vi "json Parse core.vi"(8 "error in (no error)":errorcluster, 9 "default":variant, 10 "path":string, 11 "JSON Document in":refnum<class "JSON Document.lvclass">) -> (0 "error out":errorcluster, 1 "defaulted paths":string[](array[string]), 2 "value":variant, 3 "JSON Document out":refnum<class "JSON Document.lvclass">)   [LabVIEW 2016, in "JSON Document.lvclass"]
uses:
  JSON Document.lvclass
  <vilib>/Utility/Data Type/NI_Data Type.lvlib
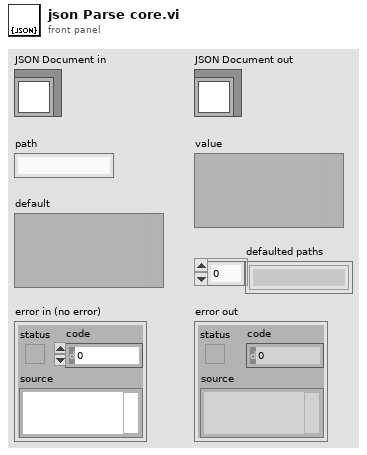
[diagram p1: front panel]
types:
  T1 = typedef "NI_Data Type.lvlib/Data Type.ctl" = enum8{"Invalid Type", "Void", "I8", "I16", "I32", "I64", "U8", "U16", "U32", "U64", "Single Float", "Double Float", "Extended Float", "Single Complex", "Double Complex", "Extended Complex", "Enum U8", "Enum U16", "Enum U32", "Enum U64", "Single Float With Unit", "Double Float With Unit", "Extended Float With Unit", "Single Complex with Unit", "Double Complex with Unit", "Extended Complex with Unit", "Boolean", "String", "Path", "Picture", "Tag", "Array", "Cluster", "Variant", "LV Variant", "Waveform", "Timestamp", "Digital Waveform", "Digital Data", "ExpressData", "Refnum", "External Data", "VI", "Poly VI", "LabVIEW Class Instance", "Fixed Point"}
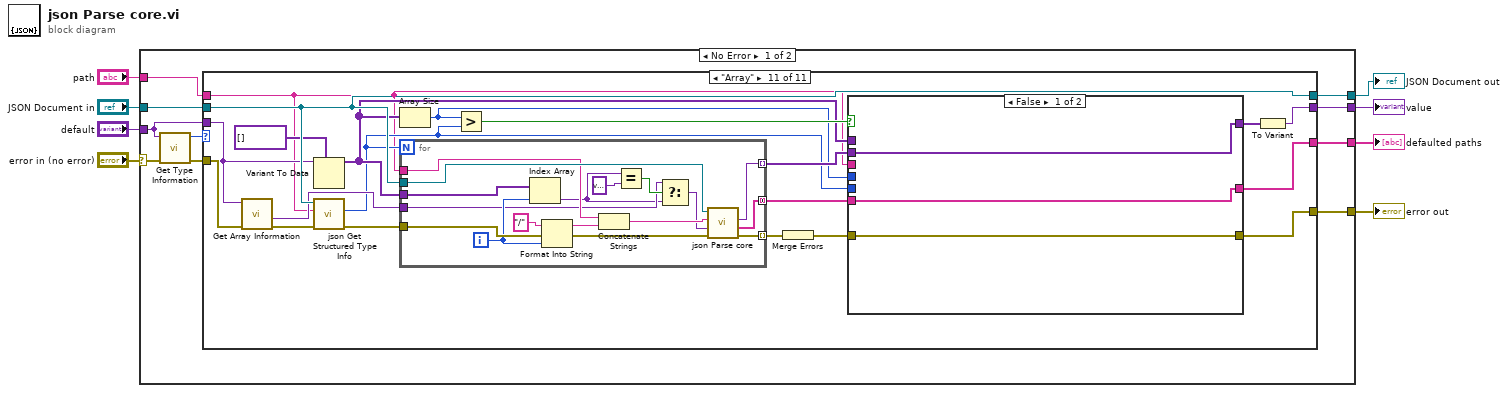
[diagram p0: block diagram]
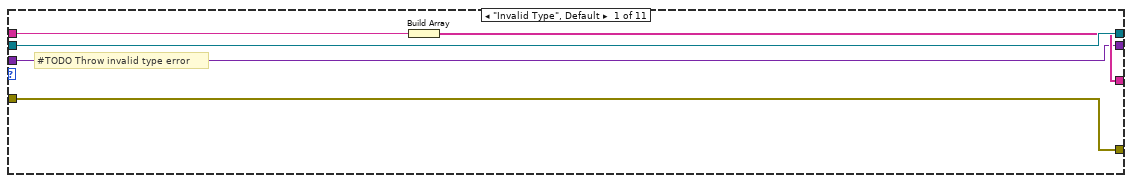
[diagram p2: hidden frame]
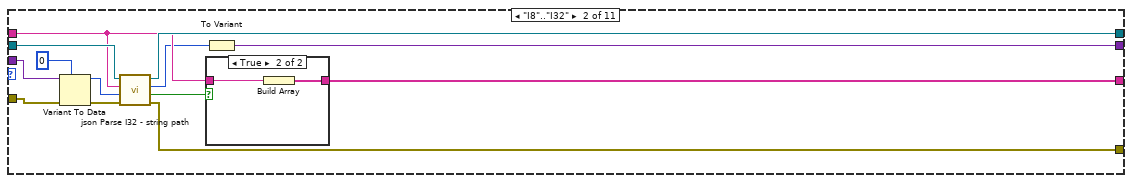
[diagram p3: hidden frame]
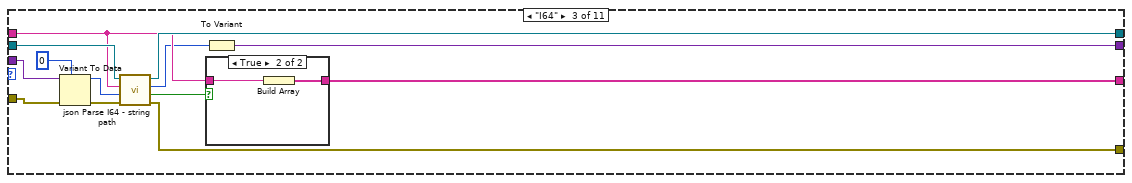
[diagram p5: hidden frame]
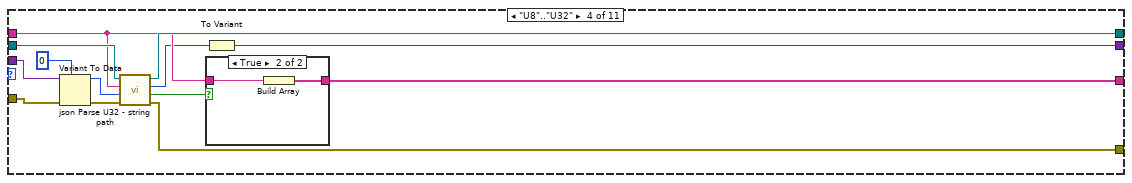
[diagram p7: hidden frame]
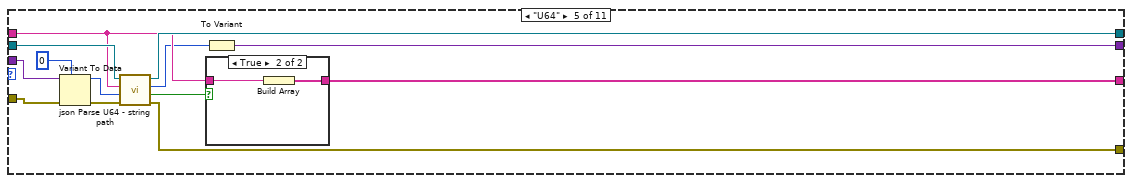
[diagram p9: hidden frame]
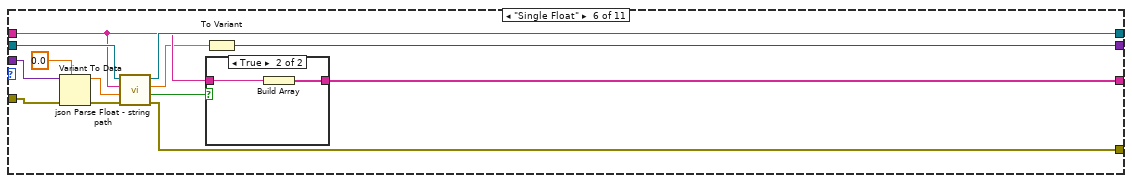
[diagram p11: hidden frame]
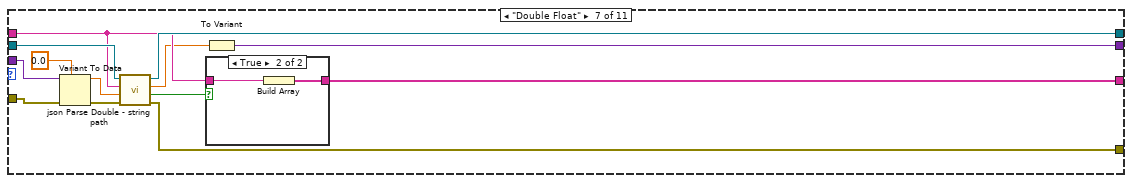
[diagram p13: hidden frame]
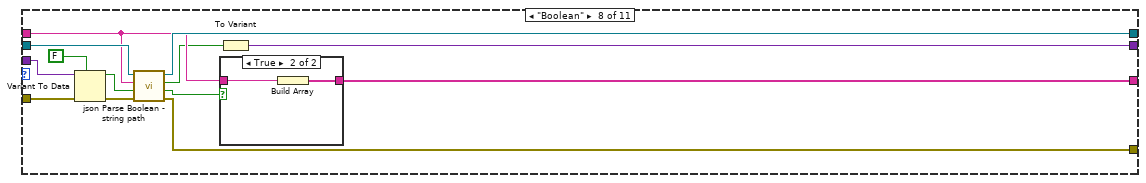
[diagram p15: hidden frame]
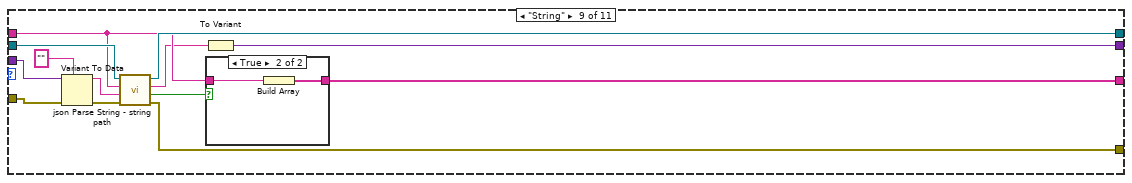
[diagram p17: hidden frame]
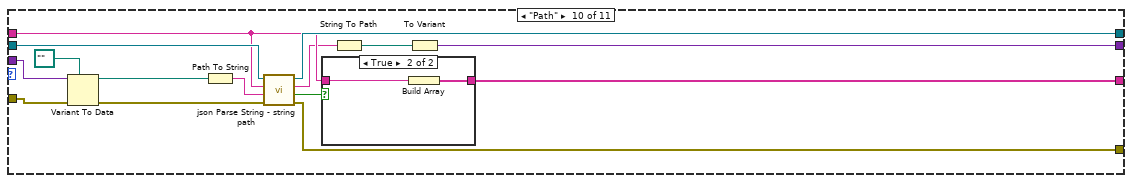
[diagram p19: hidden frame]
diagram:
  n1 = case shown="No Error" "error in (no error)" {
    selector: "error in (no error)" -> [w17 w224]
    tunnel: "JSON Document in" -> [w15 w225]
    tunnel: "default" -> [w13 w228]
    tunnel: "path" -> [w16 w227]
    tunnel: [w14 w225] -> w4
    tunnel: [w11 w224] -> w3
    tunnel: [w10 w226] -> w2
    tunnel: [w9 w228] -> w1
    frame No Error {
      n2 = call <vilib>:"Get Type Information.vi"("error in (no error)"=w17, "Variant"=w13) -> ("error out"=w12:errorcluster, "Type"=w18:T1)  [unwired: 5 in, 3 out]
      n3 = case shown="\"Array\"" w18 {
        tunnel: w16 -> [w21 w27 w42 w57 w72 w87 w102 w117 w132 w150 w165]
        tunnel: w15 -> [w23 w36 w51 w66 w81 w96 w111 w126 w141 w158 w178]
        tunnel: [w23 w35 w50 w65 w80 w95 w110 w125 w140 w157 w178] -> w14
        tunnel: w13 -> [w19 w33 w48 w63 w78 w93 w108 w123 w138 w155 w173]
        tunnel: w12 -> [w22 w32 w47 w62 w77 w92 w107 w122 w137 w154 w176]
        tunnel: [w22 w29 w44 w59 w74 w89 w104 w119 w134 w152 w161] -> w11
        tunnel: [w20 w26 w41 w56 w71 w86 w101 w116 w131 w149 w163] -> w10
        tunnel: [w19 w24 w39 w54 w69 w84 w99 w114 w129 w148 w177] -> w9
        frame "Invalid Type", Default {
          # "#TODO Throw invalid type error"
          n4 = Build Array(w21) -> (w20:string[])
        }
        frame "I8".."I32" {
          n5 = Variant To Data(error in=w32, type=0, Variant=w33) -> (data=w31:i32, error out=w30:errorcluster)
          n6 = call "json Parse I32 - string path.vi"("error in (no error)"=w30, "default"=w31, "path"=w27, "JSON Document in"=w36) -> ("error out"=w29:errorcluster, "defaulted?"=w28:bool, "value"=w25:i32, "JSON Document out"=w35:refnum<class "JSON Document.lvclass">)  [unwired: 4 in]
          n7 = case shown="True" w28 {
            tunnel: w27 -> [_ w38]
            tunnel: [_ w37] -> w26
            frame False {
            }
            frame True {
              n8 = Build Array(w38) -> (w37:string[])
            }
          }
          n9 = To Variant(anything=w25) -> (Variant=w24:variant)
        }
        frame "I64" {
          n10 = Variant To Data(error in=w47, type=i64 0, Variant=w48) -> (data=w46:i64, error out=w45:errorcluster)
          n11 = call "json Parse I64 - string path.vi"("error in (no error)"=w45, "default"=w46, "path"=w42, "JSON Document in"=w51) -> ("error out"=w44:errorcluster, "defaulted?"=w43:bool, "value"=w40:i64, "JSON Document out"=w50:refnum<class "JSON Document.lvclass">)  [unwired: 4 in]
          n12 = case shown="True" w43 {
            tunnel: w42 -> [_ w53]
            tunnel: [_ w52] -> w41
            frame False {
            }
            frame True {
              n13 = Build Array(w53) -> (w52:string[])
            }
          }
          n14 = To Variant(anything=w40) -> (Variant=w39:variant)
        }
        frame "U8".."U32" {
          n15 = Variant To Data(error in=w62, type=u32 0, Variant=w63) -> (data=w61:u32, error out=w60:errorcluster)
          n16 = call "json Parse U32 - string path.vi"("error in (no error)"=w60, "default"=w61, "path"=w57, "JSON Document in"=w66) -> ("error out"=w59:errorcluster, "defaulted?"=w58:bool, "value"=w55:u32, "JSON Document out"=w65:refnum<class "JSON Document.lvclass">)  [unwired: 4 in]
          n17 = case shown="True" w58 {
            tunnel: w57 -> [_ w68]
            tunnel: [_ w67] -> w56
            frame False {
            }
            frame True {
              n18 = Build Array(w68) -> (w67:string[])
            }
          }
          n19 = To Variant(anything=w55) -> (Variant=w54:variant)
        }
        frame "U64" {
          n20 = Variant To Data(error in=w77, type=u64 0, Variant=w78) -> (data=w76:u64, error out=w75:errorcluster)
          n21 = call "json Parse U64 - string path.vi"("error in (no error)"=w75, "default"=w76, "path"=w72, "JSON Document in"=w81) -> ("error out"=w74:errorcluster, "defaulted?"=w73:bool, "value"=w70:u64, "JSON Document out"=w80:refnum<class "JSON Document.lvclass">)  [unwired: 4 in]
          n22 = case shown="True" w73 {
            tunnel: w72 -> [_ w83]
            tunnel: [_ w82] -> w71
            frame False {
            }
            frame True {
              n23 = Build Array(w83) -> (w82:string[])
            }
          }
          n24 = To Variant(anything=w70) -> (Variant=w69:variant)
        }
        frame "Single Float" {
          n25 = Variant To Data(error in=w92, type=sgl 0.0, Variant=w93) -> (data=w91:sgl, error out=w90:errorcluster)
          n26 = call "json Parse Float - string path.vi"("error in (no error)"=w90, "default"=w91, "path"=w87, "JSON Document in"=w96) -> ("error out"=w89:errorcluster, "defaulted?"=w88:bool, "value"=w85:sgl, "JSON Document out"=w95:refnum<class "JSON Document.lvclass">)  [unwired: 4 in]
          n27 = case shown="True" w88 {
            tunnel: w87 -> [_ w98]
            tunnel: [_ w97] -> w86
            frame False {
            }
            frame True {
              n28 = Build Array(w98) -> (w97:string[])
            }
          }
          n29 = To Variant(anything=w85) -> (Variant=w84:variant)
        }
        frame "Double Float" {
          n30 = Variant To Data(error in=w107, type=0.0, Variant=w108) -> (data=w106:dbl, error out=w105:errorcluster)
          n31 = call "json Parse Double - string path.vi"("error in (no error)"=w105, "default"=w106, "path"=w102, "JSON Document in"=w111) -> ("error out"=w104:errorcluster, "defaulted?"=w103:bool, "value"=w100:dbl, "JSON Document out"=w110:refnum<class "JSON Document.lvclass">)  [unwired: 4 in]
          n32 = case shown="True" w103 {
            tunnel: w102 -> [_ w113]
            tunnel: [_ w112] -> w101
            frame False {
            }
            frame True {
              n33 = Build Array(w113) -> (w112:string[])
            }
          }
          n34 = To Variant(anything=w100) -> (Variant=w99:variant)
        }
        frame "Boolean" {
          n35 = Variant To Data(error in=w122, type=FALSE, Variant=w123) -> (data=w121:bool, error out=w120:errorcluster)
          n36 = call "json Parse Boolean - string path.vi"("error in (no error)"=w120, "default"=w121, "path"=w117, "JSON Document in"=w126) -> ("error out"=w119:errorcluster, "defaulted?"=w118:bool, "value"=w115:bool, "JSON Document out"=w125:refnum<class "JSON Document.lvclass">)  [unwired: 4 in]
          n37 = case shown="True" w118 {
            tunnel: w117 -> [_ w128]
            tunnel: [_ w127] -> w116
            frame False {
            }
            frame True {
              n38 = Build Array(w128) -> (w127:string[])
            }
          }
          n39 = To Variant(anything=w115) -> (Variant=w114:variant)
        }
        frame "String" {
          n40 = Variant To Data(error in=w137, type="", Variant=w138) -> (data=w136:string, error out=w135:errorcluster)
          n41 = call "json Parse String - string path.vi"("error in (no error)"=w135, "default"=w136, "path"=w132, "JSON Document in"=w141) -> ("error out"=w134:errorcluster, "defaulted?"=w133:bool, "value"=w130:string, "JSON Document out"=w140:refnum<class "JSON Document.lvclass">)  [unwired: 4 in]
          n42 = To Variant(anything=w130) -> (Variant=w129:variant)
          n43 = case shown="True" w133 {
            tunnel: w132 -> [_ w143]
            tunnel: [_ w142] -> w131
            frame False {
            }
            frame True {
              n44 = Build Array(w143) -> (w142:string[])
            }
          }
        }
        frame "Path" {
          n45 = Variant To Data(error in=w154, type=path "", Variant=w155) -> (data=w147:path, error out=w153:errorcluster)
          n46 = Path To String(path=w147) -> (string=w146:string)
          n47 = call "json Parse String - string path.vi"("error in (no error)"=w153, "default"=w146, "path"=w150, "JSON Document in"=w158) -> ("error out"=w152:errorcluster, "defaulted?"=w151:bool, "value"=w145:string, "JSON Document out"=w157:refnum<class "JSON Document.lvclass">)  [unwired: 4 in]
          n48 = case shown="True" w151 {
            tunnel: w150 -> [_ w160]
            tunnel: [_ w159] -> w149
            frame False {
            }
            frame True {
              n49 = Build Array(w160) -> (w159:string[])
            }
          }
          n50 = String To Path(string=w145) -> (path=w144:path)
          n51 = To Variant(anything=w144) -> (Variant=w148:variant)
        }
        frame "Array" {
          n52 = call <vilib>:"Get Array Information.vi"("error in (no error)"=w176, "Variant"=w173) -> ("error out"=w175:errorcluster, "Array Element Data Type"=w174:variant)  [unwired: 6 in, 2 out]
          n53 = Variant To Data(type=variant[] [], Variant=w173) -> (data=w170:variant[])  [unwired: 1 in, 1 out]
          n54 = call "json Get Structured Type Info.vi"("error in (no error)"=w175, "path"=w165, "JSON Document in"=w178) -> ("error out"=w180:errorcluster, "count"=w166:i32)  [unwired: 5 in, 2 out]
          n55 = Array Size(array=w170) -> (size(s)=w167:i32)
          n56 = for {
            N: w166 -> [_]
            tunnel: [w222] -> w179 mode=indexing
            tunnel: [w221] -> w169 mode=indexing
            tunnel: w174 -> [w209]
            tunnel: w180 -> [w219]
            tunnel: [w220] -> w164 mode=concatenating
            tunnel: w178 -> [w217]
            tunnel: w165 -> [w216]
            tunnel: w170 -> [w213]
            i -> [w212]
            n57 = Index Array(array=w213, index=w212) -> (element=w208:variant)
            n58 = Format Into String(initial string="/", error in=w219, w212) -> (resulting string=w215:string, error out=w218:errorcluster)  [unwired: 1 in]
            n59 = Concatenate Strings(w216, w215) -> (w214:string)
            n60 = Equal?(x=w208, y=variant) -> (x = y?=w210:bool)
            n61 = Select(t=w209, s=w210, f=w208) -> (s? t:f=w207:variant)
            n62 = call "json Parse core.vi"("error in (no error)"=w218, "default"=w207, "path"=w214, "JSON Document in"=w217) -> ("error out"=w222:errorcluster, "defaulted paths"=w220:string[], "value"=w221:variant)  [unwired: 4 in, 1 out]
          }
          n63 = Greater?(x=w167, y=w166) -> (0:w171:bool)
          n64 = Merge Errors(w179) -> (w162:errorcluster)
          n65 = case shown="False" w171 {
            tunnel: w170 -> [_ w197]
            tunnel: w169 -> [w183 w196]
            tunnel: [w183 w194] -> w168
            tunnel: w167 -> [_ w193]
            tunnel: w166 -> [_ w191]
            tunnel: w165 -> [_ w190]
            tunnel: w164 -> [w182 w189]
            tunnel: [w182 w187] -> w163
            tunnel: w162 -> [w181 w186]
            tunnel: [w181 w184] -> w161
            frame False {
            }
            frame True {
              n66 = Subtract(x=w193, y=w191) -> (x-y=w192:i32)
              n67 = Replace Array Subset(array=w197, new element=w196, index=0) -> (w194:variant[])
              n68 = for {
                N: w192 -> [_]
                tunnel: w191 -> [w206]
                tunnel: w190 -> [w202]
                tunnel: [w200] -> w188 mode=indexing
                tunnel: w186 -> [w199]
                tunnel: [w198] -> w185 mode=indexing
                i -> [w205]
                n69 = Add(x=w206, y=w205) -> (x+y=w203:i32)
                n70 = Format Into String(initial string="/", error in=w199, w203) -> (resulting string=w201:string, error out=w198:errorcluster)  [unwired: 1 in]
                n71 = Concatenate Strings(w202, w201) -> (w200:string)
              }
              n72 = Build Array (concatenate)(w189, w188) -> (w187:string[])
              n73 = Merge Errors(w185) -> (w184:errorcluster)
            }
          }
          n74 = To Variant(anything=w168) -> (Variant=w177:variant)
        }
      }
    }
    frame Error {
      n75 = Build Array(w227) -> (w226:string[])
    }
  }
  "error out" <- w3
  "JSON Document out" <- w4
  "value" <- w1
  "defaulted paths" <- w2
